vi "GetTableLoggerConfig.vi"(8 "error in (no error)":errorcluster, 11 "object in":refnum<class "TableLogger_Actor.lvclass">) -> (0 "error out":errorcluster, 2 "TableLogger Config":T1, 3 "object out":refnum<class "TableLogger_Actor.lvclass">)   [LabVIEW 2014, in "TableLogger_Actor.lvlib" / "TableLogger_Actor.lvclass"]
uses:
  TableLogger_Actor.lvclass
  TableLoggerConfig.ctl
  TableLoggerTypes.ctl
  TableLoggerBackupConfig.ctl
  TableLogger_Actor.lvclass/TableLogger_Actor.ctl
  TableLogger_Actor.lvlib
panel:
  # "Connector Pane"
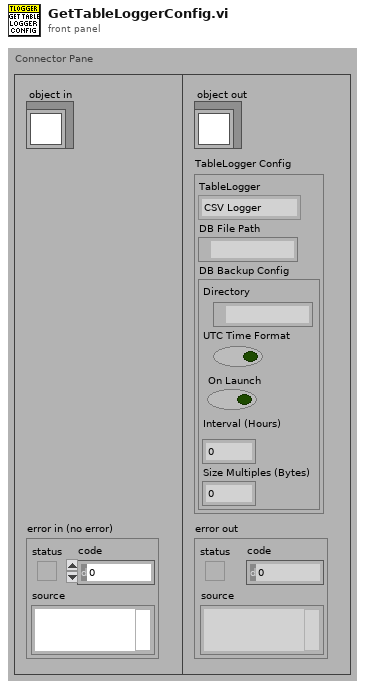
[diagram p1: front panel]
types:
  T1 = typedef "TableLogger_Actor.lvlib/TableLoggerConfig.ctl" = cluster{"TableLogger":T2, "DB File Path":path, "DB Backup Config":T3}
  T2 = typedef "TableLogger_Actor.lvlib/TableLoggerTypes.ctl" = enum16{"CSV Logger", "SQLite Logger"}
  T3 = typedef "TableLogger_Actor.lvlib/TableLoggerBackupConfig.ctl" = cluster{"Directory":path, "UTC Time Format":bool, "On Launch":bool, "Interval (Hours)":dbl, "Size Multiples (Bytes)":i32}
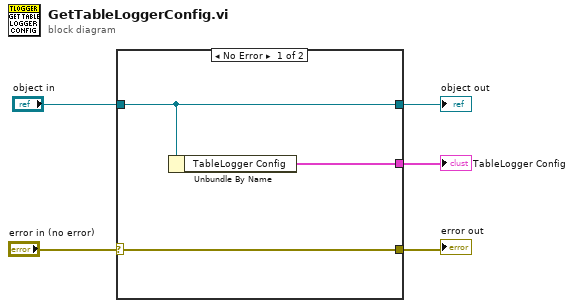
[diagram p0: block diagram]
diagram:
  n1 = case shown="No Error" "error in (no error)" {
    selector: "error in (no error)" -> [w7 w10]
    tunnel: [w7 w10] -> w4
    tunnel: [w6 w9] -> w2
    tunnel: "object in" -> [w6 w9]
    tunnel: [w8 _] -> w1
    frame No Error {
      n2 = Unbundle By Name(w6) -> ("TableLogger Config"=w8:T1)
    }
    frame Error {
    }
  }
  "error out" <- w4
  "object out" <- w2
  "TableLogger Config" <- w1
